vi "Handle TCP Message.vi"(7 "TCPMessageAPI":refnum<class "TCPMessageAPI.lvclass">, 8 "error in (no error)":errorcluster, 10 "TcpPayload":T1, 11 "Simple TCP Handler in":refnum<class "Simple TCP Handler.lvclass">) -> (0 "error out":errorcluster, 3 "Simple TCP Handler out":refnum<class "Simple TCP Handler.lvclass">)   [LabVIEW 2020, in "VectoScratch.lvlib" / "Simple TCP Handler.lvclass"]
uses:
  Simple TCP Handler.lvclass
  Vecto/TCPMessageService/TCPMessageAPI.lvclass
  Vecto/proto/TcpPayload/Data.ctl
  Simple TCP Handler.lvclass/Simple TCP Handler.ctl
  Vecto/proto/TcpPayload/TcpPayload.lvlib
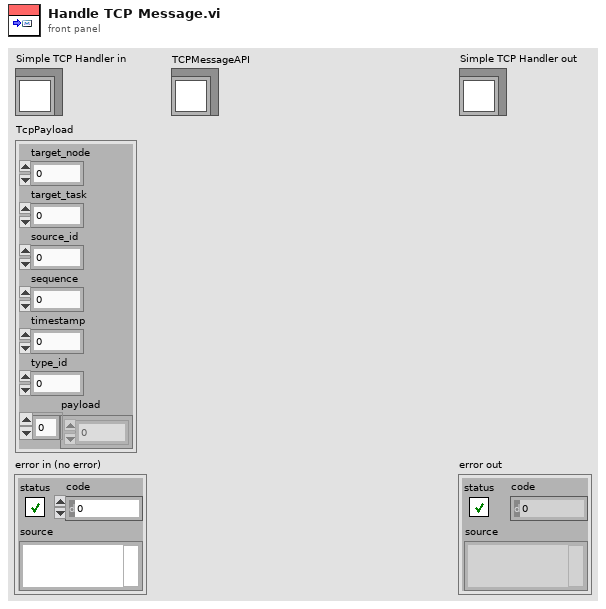
[diagram p1: front panel]
types:
  T1 = typedef "TcpPayload.lvlib/Data.ctl" = cluster{"target_node":u32, "target_task":u32, "source_id":u32, "sequence":u32, "timestamp":u64, "type_id":u32, "payload":u8[]}
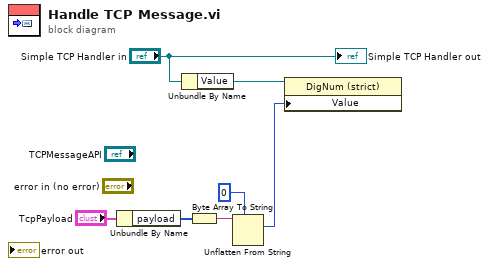
[diagram p0: block diagram]
diagram:
  n1 = Unbundle By Name("TcpPayload") -> ("payload"=w1:u8[])
  n2 = Unbundle By Name("Simple TCP Handler in") -> ("Value"=w6:refnum<vi>)
  n3 = Byte Array To String(unsigned byte array=w1) -> (string=w2:string)
  n4 = Unflatten From String(type=0, binary string=w2) -> (value=w4:i32)  [unwired: 3 in, 2 out]
  n5 = property class="DigNum (strict)"(reference=w6, "Value"=w4) -> ()  [unwired: 1 in, 2 out]
  "Simple TCP Handler out" <- "Simple TCP Handler in"
